vi "Read Scale Icon.vi"(8 "error in (no error)":errorcluster, 11 "Control in":refnum<class "Control.lvclass">) -> (0 "error out":errorcluster, 2 "Scale Icon":dbl(slide)=1.0 min=0.25 max=5.0 scale=0.25..5.0, 3 "Control out":refnum<class "Control.lvclass">)   [LabVIEW 2013, in "uitools_Control.lvlib" / "Control.lvclass"]
uses:
  Control.lvclass
  Control.lvclass/Control.ctl
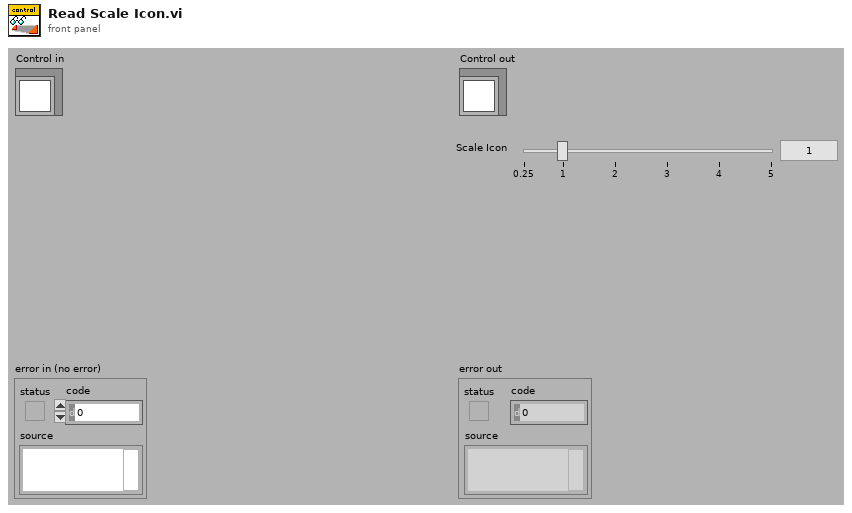
[diagram p1: front panel]
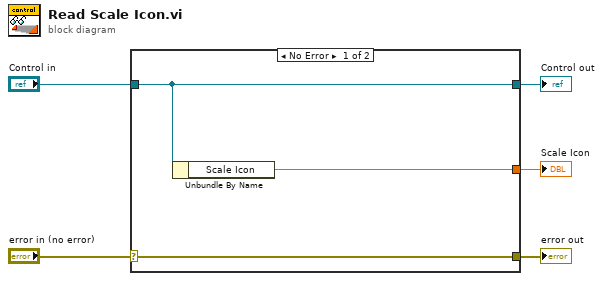
[diagram p0: block diagram]
diagram:
  n1 = case shown="No Error" "error in (no error)" {
    selector: "error in (no error)" -> [w8 w9]
    tunnel: [w8 w9] -> w4
    tunnel: [w7 w10] -> w2
    tunnel: "Control in" -> [w7 w10]
    tunnel: [w6 _] -> w1
    frame No Error {
      n2 = Unbundle By Name(w7) -> ("Scale Icon"=w6:dbl)
    }
    frame Error {
    }
  }
  "error out" <- w4
  "Control out" <- w2
  "Scale Icon" <- w1
